vi "Circle2004.vi"   [LabVIEW 2013]
uses:
  <vilib>/Heliosphere Research LLC/Advanced Plotting Toolkit/api_core/NewPlotProperties.ctl
  <vilib>/Heliosphere Research LLC/Advanced Plotting Toolkit/typedefs/PlotColor.ctl
  <vilib>/Heliosphere Research LLC/Advanced Plotting Toolkit/Advanced Plotting Toolkit.lvlib
types:
  T1 = typedef "Advanced Plotting Toolkit.lvlib/NewPlotProperties.ctl" = cluster{"Background Color":T2, "Axis Background":T2, "Left Margin":dbl, "Right Margin":dbl, "Bottom Margin":dbl, "Top Margin":dbl, "Aspect Ratio":dbl}
  T2 = typedef "Advanced Plotting Toolkit.lvlib/PlotColor.ctl" = u32
  T3 = typedef "Advanced Plotting Toolkit.lvlib/PlotID.ctl" = i32
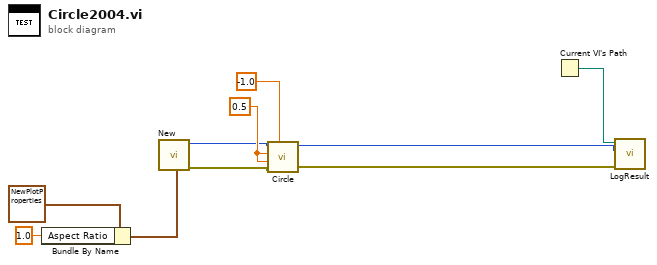
[diagram p0: block diagram]
diagram:
  w9 = 0.5 ("X Position")
  n1 = Bundle By Name(cluster=T1 {"Background Color"=2147483647, "Axis Background"=2147483647, "Left Margin"=nan, "Right Margin"=nan, "Bottom Margin"=nan, "Top Margin"=nan, "Aspect Ratio"=nan} ("New Plot Properties"), "Aspect Ratio"=1.0) -> (w3:T1)
  n2 = call <vilib>:"New.vi"("Properties"=w3) -> ("error out"=w7:errorcluster, "Plot ID"=w8:T3)  [unwired: 9 in]
  n3 = call <vilib>:"Circle.vi"("Radius"=-1.0, "error in (no error)"=w7, "Y Position"=w9, "X Position"=w9, "Plot ID"=w8) -> ("error out"=w5:errorcluster, "Plot ID Out"=w6:T3)  [unwired: 5 in]
  n4 = Current VI's Path() -> (path=w10:path)
  n5 = call "LogResult.vi"("Test Result"=w5, "Test Artifact"=w6, "VI Path"=w10) -> ()  [unwired: 9 in]
